vi "trayectoriasQuintoOrden.vi"(8 "tf":dbl, 9 "thetaf":dbl, 10 "thetai":dbl) -> (0 "a4":dbl, 1 "a3":dbl, 2 "a2":dbl, 3 "a1":dbl, 4 "a5":dbl, 5 "a0":dbl)   [LabVIEW 2019]
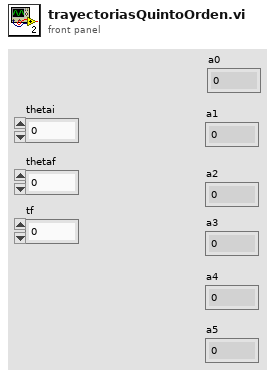
[diagram p1: front panel]
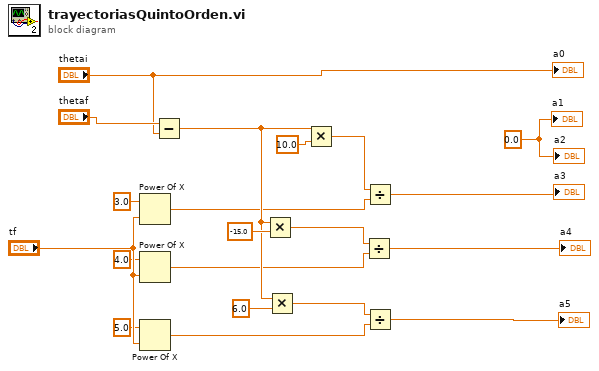
[diagram p0: block diagram]
diagram:
  w20 = 0.0 ("a1")
  n1 = Power Of X(1:"tf", 2:3.0 ("y")) -> (0:w10:dbl)
  n2 = Power Of X(1:"tf", 2:4.0 ("y")) -> (0:w8:dbl)
  n3 = Power Of X(1:"tf", 2:5.0 ("y")) -> (0:w5:dbl)
  n4 = Subtract(x="thetaf", y="thetai") -> (x-y=w14:dbl)
  n5 = Multiply(x=w14, y=-15.0) -> (x*y=w9:dbl)
  n6 = Multiply(x=w14, y=6.0) -> (x*y=w6:dbl)
  n7 = Multiply(x=w14, y=10.0) -> (x*y=w11:dbl)
  n8 = Divide(x=w9, y=w8) -> (x/y=→"a4":dbl)
  n9 = Divide(x=w11, y=w10) -> (x/y=→"a3":dbl)
  n10 = Divide(x=w6, y=w5) -> (x/y=→"a5":dbl)
  "a0" <- "thetai"
  "a2" <- w20
  "a1" <- w20
